vi "CmdParse_3.vi"(8 "error in (no error)":errorcluster, 9 "Read Buffer":string, 10 "Node Id":u8, 11 "Socket Id":u8) -> (0 "error out":errorcluster)   [LabVIEW 2011]
uses:
  Enumerator/CmdType.ctl
  Variable/gSIM.vi
  DLL/Certificate_03.vi
  Variable/gSEL.vi
  Look-up/Password/PSW_03.vi
  Queue/Door_03.vi
  Interface/SockeHook/Hook_03.vi
panel:
  in  "KeyPass":bool
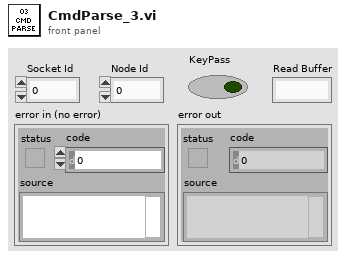
[diagram p1: front panel]
types:
  T1 = enum16{"Open", "R", "W", "R->W", "W->R", "Close"}
  T2 = typedef "CmdType.ctl" = enum16{"GetEventLog", "DelTransaction", "InvalidMessage", "RelayControl", "RelayOff", "RelayOn", "VaildMessage", "EventPolling", "StoppingWaiting", "PromptKeying-in"}
  T3 = enum16{"Open", "Verify", "Password", "Log", "Close"}
  T4 = enum16{"Obtain", "Enqueue", "Dequeue", "Release"}
  T5 = cluster{"unsigned byte array":u8[], "Socket Id":u8, u8}
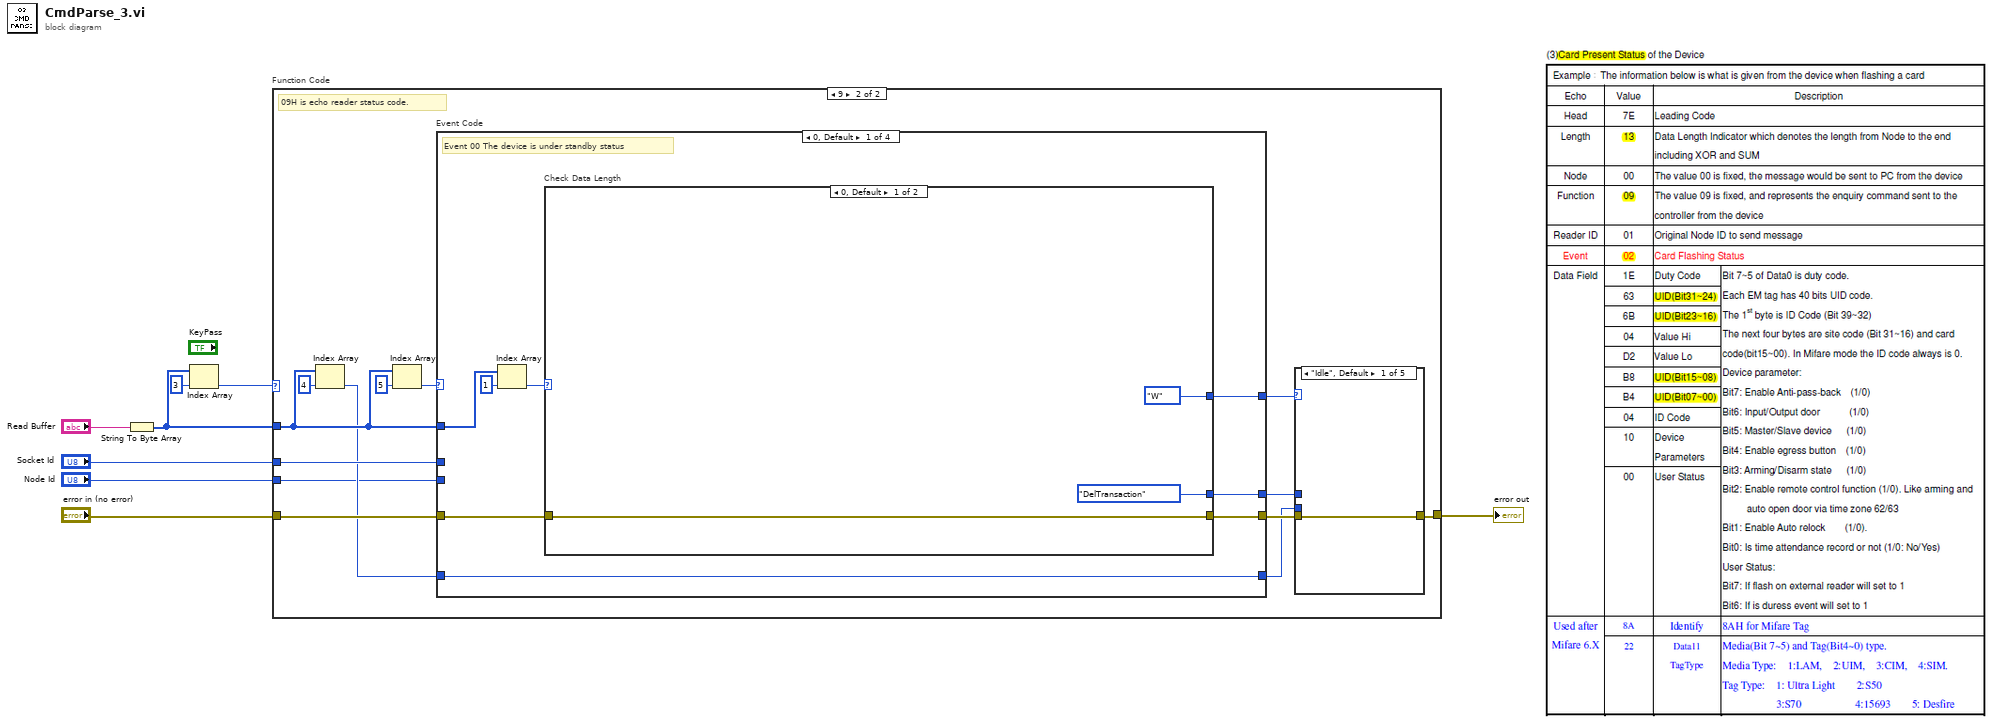
[diagram p0: block diagram]
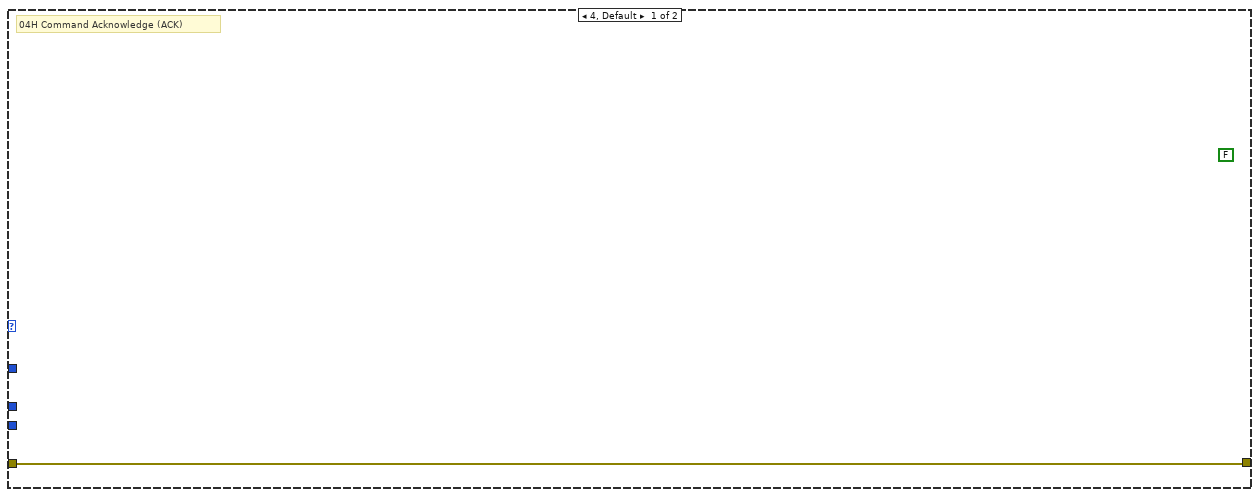
[diagram p2: hidden frame]
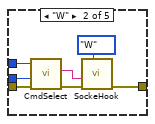
[diagram p3: hidden frame]
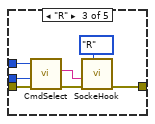
[diagram p4: hidden frame]
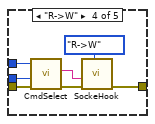
[diagram p5: hidden frame]
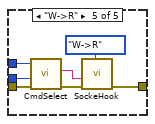
[diagram p6: hidden frame]
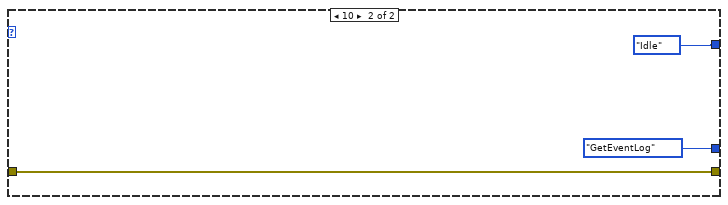
[diagram p7: hidden frame]
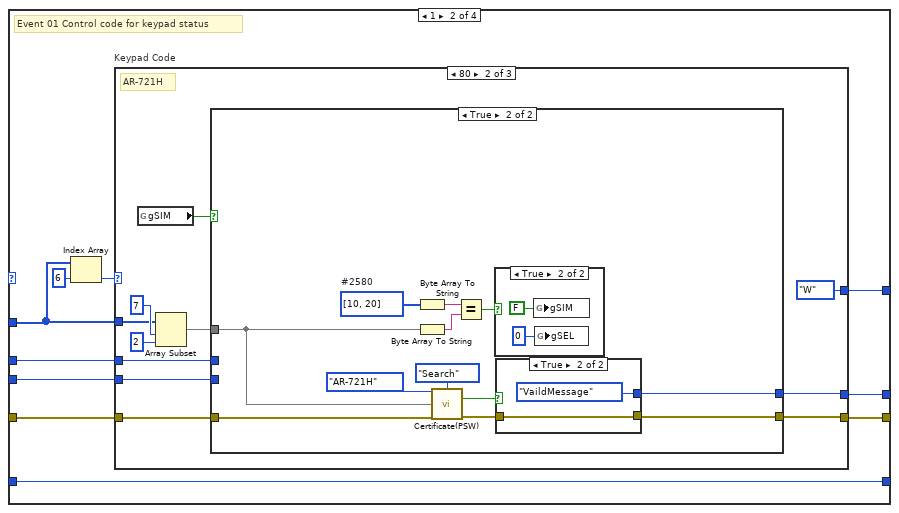
[diagram p8: hidden frame]
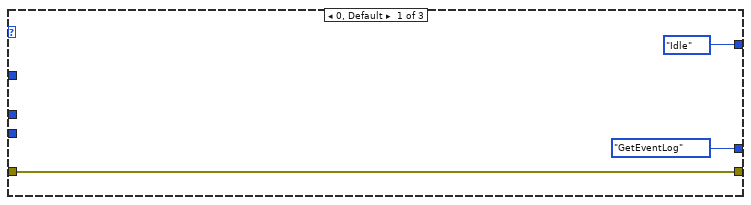
[diagram p9: hidden frame]
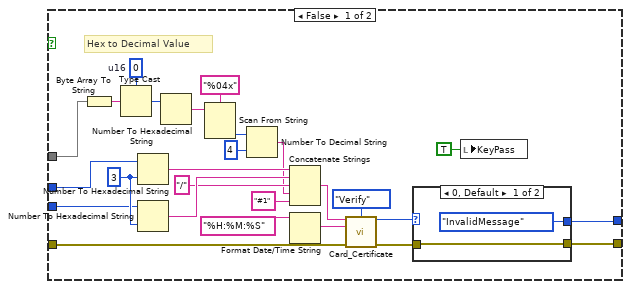
[diagram p10: hidden frame]
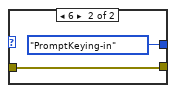
[diagram p11: hidden frame]
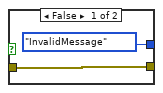
[diagram p12: hidden frame]
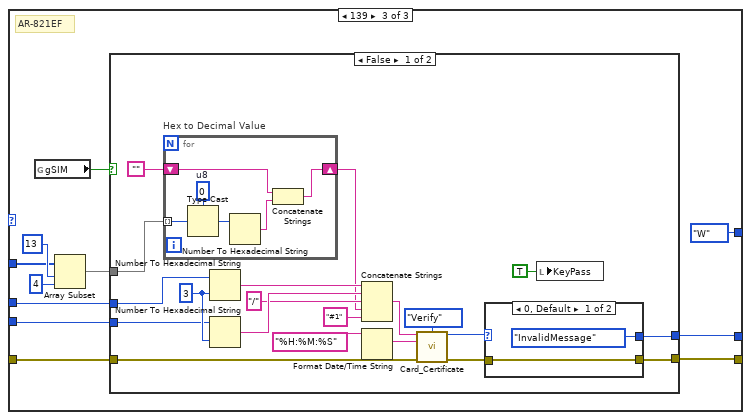
[diagram p14: hidden frame]
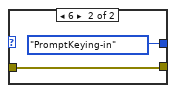
[diagram p15: hidden frame]
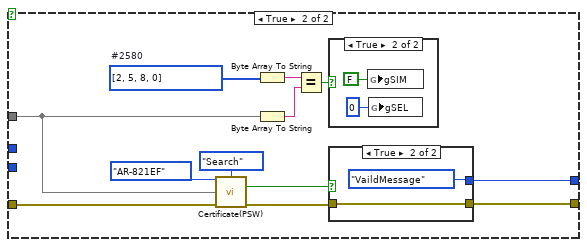
[diagram p16: hidden frame]
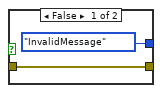
[diagram p17: hidden frame]
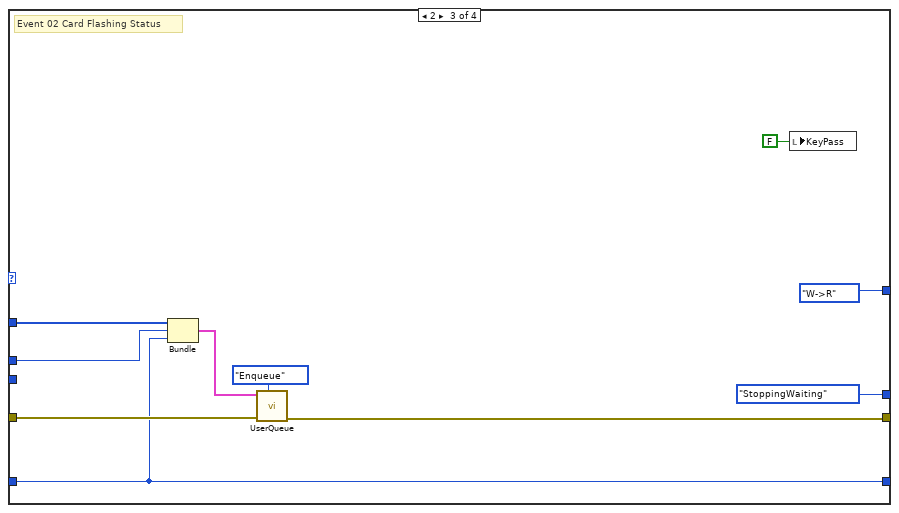
[diagram p19: hidden frame]
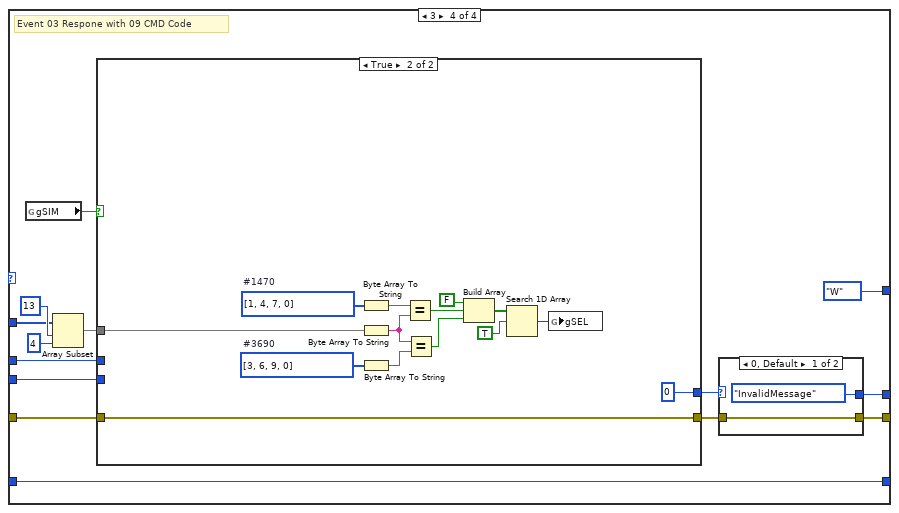
[diagram p20: hidden frame]
diagram:
  n1 = String To Byte Array(string="Read Buffer") -> (unsigned byte array=w2:u8[])
  n2 = Index Array(array=w2, index=3) -> (element=w5:u8)
  n3 = case "Function Code" shown="9" w5 {
    tunnel: "error in (no error)" -> [w9 w22]
    tunnel: [w9 w14] -> w8
    tunnel: w2 -> [_ w20]
    tunnel: "Socket Id" -> [_ w19]
    tunnel: "Node Id" -> [_ w10]
    frame 4, Default {
      (unwired) FALSE
      # "04H Command Acknowledge (ACK)"
    }
    frame 9 {
      # "09H is echo reader status code."
      n4 = Index Array(array=w20, index=4) -> (element=w16:u8)
      n5 = Index Array(array=w20, index=5) -> (element=w17:u8)
      n6 = case "Event Code" shown="0, Default" w17 {
        tunnel: w22 -> [w59 w75 w199 w212]
        tunnel: w16 -> [w52 w68 w198 w216]
        tunnel: [w58 w74 w206 w218] -> w15
        tunnel: w20 -> [w55 w71 w204 w215]
        tunnel: w19 -> [_ w67 w203 w208]
        tunnel: [w52 w68 w198 w216] -> w13
        tunnel: [w54 w70 CmdType."StoppingWaiting" ("CmdType") w214] -> w12
        tunnel: [w53 w69 enum16{"Idle", "R", "W", "R->W", "W->R"}."W->R" ("Mode") enum16{"Idle", "R", "W", "R->W", "W->R"}."W" ("Mode")] -> w11
        tunnel: w10 -> [_ w66 _ w207]
        frame 0, Default {
          # "Event 00 The device is under standby status"
          n7 = Index Array(array=w55, index=1) -> (element=w56:u8)
          n8 = case "Check Data Length" shown="0, Default" w56 {
            tunnel: w59 -> [w62 w65]
            tunnel: [w62 w65] -> w58
            tunnel: [CmdType."DelTransaction" ("CmdType") CmdType."GetEventLog" ("CmdType")] -> w54
            tunnel: [enum16{"Idle", "R", "W", "R->W", "W->R"}."W" ("Mode") enum16{"Idle", "R", "W", "R->W", "W->R"}."Idle" ("Mode")] -> w53
            frame 0, Default {
            }
            frame 10 {
            }
          }
        }
        frame 1 {
          # "Event 01 Control code for keypad status"
          n9 = Index Array(array=w71, index=6) -> (element=w72:u8)
          n10 = case "Keypad Code" shown="80" w72 {
            tunnel: w75 -> [w78 w82 w142]
            tunnel: [w78 w83 w141] -> w74
            tunnel: w71 -> [_ w87 w146]
            tunnel: [CmdType."GetEventLog" ("CmdType") w81 w140] -> w70
            tunnel: [enum16{"Idle", "R", "W", "R->W", "W->R"}."Idle" ("Mode") enum16{"Idle", "R", "W", "R->W", "W->R"}."W" ("Mode") enum16{"Idle", "R", "W", "R->W", "W->R"}."W" ("Mode")] -> w69
            tunnel: w67 -> [_ w80 w139]
            tunnel: w66 -> [_ w79 w138]
            frame 0, Default {
            }
            frame 128 {
              # "AR-721H"
              n11 = global read "gSIM.vi" "gSIM"() -> (w85:bool)
              n12 = Array Subset(array=w87, index=7, length=2) -> (w84:u8[])
              n13 = case shown="True" w85 {
                tunnel: w84 -> [w98 w120]
                tunnel: [w113 w123] -> w83
                tunnel: w82 -> [w114 w122]
                tunnel: [w110 w121] -> w81
                tunnel: w80 -> [w103 _]
                tunnel: w79 -> [w102 _]
                frame False {
                  w97 = u16 0  # u16
                  w106 = i16 3 ("width (-)")
                  # "Hex to Decimal Value"
                  n14 = Byte Array To String(unsigned byte array=w98) -> (string=w99:string)
                  n15 = Type Cast(type=w97, x=w99) -> (*(type *) &x=w96:u16)
                  n16 = Number To Hexadecimal String(1:w106, 2:w103) -> (0:w109:string)
                  n17 = Number To Hexadecimal String(1:w106, 2:w102) -> (0:w108:string)
                  n18 = Number To Hexadecimal String(2:w96) -> (0:w95:string)  [unwired: 1 in]
                  n19 = Scan From String(format string="%04x", input string=w95) -> (output 1=w93:i32)  [unwired: 2 in, 4 out]
                  n20 = Number To Decimal String(number=w93, width (-)=i16 4) -> (decimal integer string=w92:string)
                  n21 = Concatenate Strings(w109, w108, "/" ("string"), w92, "#1" ("string")) -> (w100:string)
                  n22 = Format Date/Time String(time format string (%c)="%H:%M:%S") -> (date/time string=w101:string)  [unwired: 2 in]
                  n23 = call-poly "Card_Certificate.vi"("CardNumber"=w100, "DB"=T3."Verify", "Time"=w101, "error in"=w114) -> ("Certificate"=w111:u8, "error out"=w112:errorcluster)  [unwired: 10 in]
                  n24 = case shown="0, Default" w111 {
                    tunnel: w112 -> [w117 w119]
                    tunnel: [w117 w119] -> w113
                    tunnel: [CmdType."InvalidMessage" ("CmdType") CmdType."PromptKeying-in" ("CmdType")] -> w110
                    frame 0, Default {
                    }
                    frame 6 {
                    }
                  }
                  n25 = local write "KeyPass"(TRUE ("KeyPass")) -> ()
                }
                frame True {
                  w130 = u8[] [10, 20]  # #2580
                  n26 = Byte Array To String(unsigned byte array=w130) -> (string=w131:string)
                  n27 = Byte Array To String(unsigned byte array=w120) -> (string=w129:string)
                  n28 = call-poly "Certificate(PSW).vi"("type"=enum16{"AR-721H", "AR-821EF"}."AR-721H", "select"=enum16{"Setup", "Search", "Release"}."Search", "key"=w120, "error in"=w122) -> ("found"=w127:bool, "error out"=w126:errorcluster)  [unwired: 9 in, 1 out]
                  n29 = Equal?(x=w131, y=w129) -> (x = y?=w128:bool)
                  n30 = case shown="True" w128 {
                    frame False {
                    }
                    frame True {
                      n31 = global write "gSIM.vi" "gSIM"(FALSE ("gSIM")) -> ()
                      n32 = global write "gSEL.vi" "gSEL"(0 ("gSEL")) -> ()
                    }
                  }
                  n33 = case shown="True" w127 {
                    tunnel: w126 -> [w133 w135]
                    tunnel: [w133 w135] -> w123
                    tunnel: [CmdType."InvalidMessage" ("CmdType") CmdType."VaildMessage" ("CmdType")] -> w121
                    frame False {
                    }
                    frame True {
                    }
                  }
                }
              }
            }
            frame 139 {
              # "AR-821EF"
              n34 = global read "gSIM.vi" "gSIM"() -> (w144:bool)
              n35 = Array Subset(array=w146, index=13, length=4) -> (w143:u8[])
              n36 = case shown="False" w144 {
                tunnel: w143 -> [w158 w179]
                tunnel: w142 -> [w154 w182]
                tunnel: [w162 w181] -> w141
                tunnel: [w156 w180] -> w140
                tunnel: w139 -> [w161 _]
                tunnel: w138 -> [w160 _]
                frame False {
                  w165 = i16 3 ("width (-)")
                  n37 = for "Hex to Decimal Value" {
                    shift-right: [w171] -> w157
                    shift-left: "" -> [w170]
                    tunnel: w158 -> [w169] mode=indexing
                    w173 = u8 0  # u8
                    n38 = Type Cast(type=w173, x=w169) -> (*(type *) &x=w174:u8)
                    n39 = Number To Hexadecimal String(2:w174) -> (0:w172:string)  [unwired: 1 in]
                    n40 = Concatenate Strings(w170, w172) -> (w171:string)
                  }
                  n41 = Number To Hexadecimal String(1:w165, 2:w161) -> (0:w168:string)
                  n42 = Number To Hexadecimal String(1:w165, 2:w160) -> (0:w167:string)
                  n43 = Concatenate Strings(w168, w167, "/" ("string"), w157, "#1" ("string")) -> (w151:string)
                  n44 = Format Date/Time String(time format string (%c)="%H:%M:%S") -> (date/time string=w150:string)  [unwired: 2 in]
                  n45 = call-poly "Card_Certificate.vi"("CardNumber"=w151, "DB"=T3."Verify", "Time"=w150, "error in"=w154) -> ("Certificate"=w152:u8, "error out"=w153:errorcluster)  [unwired: 10 in]
                  n46 = case shown="0, Default" w152 {
                    tunnel: w153 -> [w176 w178]
                    tunnel: [w176 w178] -> w162
                    tunnel: [CmdType."InvalidMessage" ("CmdType") CmdType."PromptKeying-in" ("CmdType")] -> w156
                    frame 0, Default {
                    }
                    frame 6 {
                    }
                  }
                  n47 = local write "KeyPass"(TRUE ("KeyPass")) -> ()
                }
                frame True {
                  w188 = u8[] [2, 5, 8, 0]  # #2580
                  n48 = call-poly "Certificate(PSW).vi"("type"=enum16{"AR-721H", "AR-821EF"}."AR-821EF", "select"=enum16{"Setup", "Search", "Release"}."Search", "key"=w179, "error in"=w182) -> ("found"=w185:bool, "error out"=w184:errorcluster)  [unwired: 9 in, 1 out]
                  n49 = Byte Array To String(unsigned byte array=w188) -> (string=w190:string)
                  n50 = Byte Array To String(unsigned byte array=w179) -> (string=w189:string)
                  n51 = Equal?(x=w190, y=w189) -> (x = y?=w187:bool)
                  n52 = case shown="True" w187 {
                    frame False {
                    }
                    frame True {
                      n53 = global write "gSIM.vi" "gSIM"(FALSE ("gSIM")) -> ()
                      n54 = global write "gSEL.vi" "gSEL"(0 ("gSEL")) -> ()
                    }
                  }
                  n55 = case shown="True" w185 {
                    tunnel: w184 -> [w192 w194]
                    tunnel: [w192 w194] -> w181
                    tunnel: [CmdType."InvalidMessage" ("CmdType") CmdType."VaildMessage" ("CmdType")] -> w180
                    frame False {
                    }
                    frame True {
                    }
                  }
                }
              }
            }
          }
        }
        frame 2 {
          # "Event 02 Card Flashing Status"
          n56 = Bundle("unsigned byte array"=w204, "Socket Id"=w203, w198) -> (w202:T5)  [unwired: 1 in]
          n57 = call-poly "UserQueue.vi"("Mode"=T4."Enqueue", "error in (no error)"=w199, "Queue In"=w202) -> ("error out"=w206:errorcluster)  [unwired: 7 in, 1 out]
          n58 = local write "KeyPass"(FALSE) -> ()
        }
        frame 3 {
          # "Event 03 Respone with 09 CMD Code"
          n59 = global read "gSIM.vi" "gSIM"() -> (w213:bool)
          n60 = Array Subset(array=w215, index=13, length=4) -> (w209:u8[])
          n61 = case shown="True" w213 {
            tunnel: w212 -> [w227 w268]
            tunnel: [w226 w268] -> w211
            tunnel: [w225 u8 0 ("Certificate")] -> w210
            tunnel: w209 -> [w224 w267]
            tunnel: w208 -> [w223 _]
            tunnel: w207 -> [w222 _]
            frame False {
              n62 = local read "KeyPass"() -> (w221:bool)
              n63 = case shown="False" w221 {
                tunnel: w227 -> [w230 w258]
                tunnel: [w231 w257] -> w226
                tunnel: [w228 w256] -> w225
                tunnel: w224 -> [w229 w255]
                tunnel: w223 -> [_ w254]
                tunnel: w222 -> [_ w253]
                frame False {
                  n64 = for "Number To Decimal String" {
                    shift-right: [w240] -> w233
                    shift-left: "" -> [w239]
                    tunnel: w229 -> [w237] mode=indexing
                    n65 = Number To Decimal String(number=w237, width (-)=i16 1) -> (decimal integer string=w238:string)
                    n66 = Concatenate Strings(w239, w238) -> (w240:string)
                  }
                  n67 = Concatenate Strings(";" ("string"), w233) -> (w234:string)
                  n68 = call-poly "Card_Certificate.vi"("DB"=T3."Password", "Password"=w234, "error in"=w230) -> ("Certificate"=w228:u8, "error out"=w231:errorcluster)  [unwired: 11 in]
                }
                frame True {
                  w248 = i16 3 ("width (-)")
                  n69 = for "Number To Decimal String" {
                    shift-right: [w262] -> w246
                    shift-left: "" -> [w261]
                    tunnel: w255 -> [w259] mode=indexing
                    n70 = Number To Decimal String(number=w259, width (-)=i16 1) -> (decimal integer string=w260:string)
                    n71 = Concatenate Strings(w261, w260) -> (w262:string)
                  }
                  n72 = Number To Hexadecimal String(1:w248, 2:w254) -> (0:w251:string)
                  n73 = Number To Hexadecimal String(1:w248, 2:w253) -> (0:w250:string)
                  n74 = Concatenate Strings(w251, w250, "/" ("string"), w246, "#2" ("string")) -> (w243:string)
                  n75 = Format Date/Time String(time format string (%c)="%H:%M:%S") -> (date/time string=w242:string)  [unwired: 2 in]
                  n76 = call-poly "Card_Certificate.vi"("CardNumber"=w243, "DB"=T3."Verify", "Time"=w242, "error in"=w258) -> ("Certificate"=w256:u8, "error out"=w257:errorcluster)  [unwired: 10 in]
                }
              }
            }
            frame True {
              w274 = u8[] [3, 6, 9, 0]  # #3690
              w270 = u8[] [1, 4, 7, 0]  # #1470
              n77 = Byte Array To String(unsigned byte array=w270) -> (string=w273:string)
              n78 = Byte Array To String(unsigned byte array=w267) -> (string=w265:string)
              n79 = Byte Array To String(unsigned byte array=w274) -> (string=w266:string)
              n80 = Equal?(x=w273, y=w265) -> (x = y?=w272:bool)
              n81 = Equal?(x=w265, y=w266) -> (x = y?=w271:bool)
              n82 = Build Array(FALSE ("element"), w272, w271) -> (w276:bool[])
              n83 = Search 1D Array(1D array=w276, element=TRUE) -> (index of element=w275:i32)  [unwired: 1 in]
              n84 = global write "gSEL.vi" "gSEL"(w275) -> ()
            }
          }
          n85 = case shown="0, Default" w210 {
            tunnel: w211 -> [w279 w281]
            tunnel: [w279 w281] -> w218
            tunnel: [CmdType."InvalidMessage" ("CmdType") CmdType."VaildMessage" ("CmdType")] -> w214
            frame 0, Default {
            }
            frame 1 {
            }
          }
        }
      }
      n86 = case shown="\"Idle\", Default" w11 {
        tunnel: w15 -> [w23 w27 w34 w41 w48]
        tunnel: [w23 w26 w33 w40 w47] -> w14
        tunnel: w13 -> [_ w25 w32 w39 w46]
        tunnel: w12 -> [_ w24 w31 w38 w45]
        frame "Idle", Default {
        }
        frame "W" {
          n87 = call "CmdSelect.vi"("error in (no error)"=w27, "Node Id"=w25, "Cmd Type"=w24) -> ("error out"=w29:errorcluster, "Cmd Str"=w28:string)  [unwired: 7 in]
          n88 = call-poly "SockeHook.vi"("Mode"=T1."W", "error in (no error)"=w29, "data in"=w28) -> ("error out"=w26:errorcluster)  [unwired: 7 in, 1 out]
        }
        frame "R" {
          n89 = call "CmdSelect.vi"("error in (no error)"=w34, "Node Id"=w32, "Cmd Type"=w31) -> ("error out"=w36:errorcluster, "Cmd Str"=w35:string)  [unwired: 7 in]
          n90 = call-poly "SockeHook.vi"("Mode"=T1."R", "error in (no error)"=w36, "data in"=w35) -> ("error out"=w33:errorcluster)  [unwired: 7 in, 1 out]
        }
        frame "R->W" {
          n91 = call "CmdSelect.vi"("error in (no error)"=w41, "Node Id"=w39, "Cmd Type"=w38) -> ("error out"=w43:errorcluster, "Cmd Str"=w42:string)  [unwired: 7 in]
          n92 = call-poly "SockeHook.vi"("Mode"=T1."R->W", "error in (no error)"=w43, "data in"=w42) -> ("error out"=w40:errorcluster)  [unwired: 7 in, 1 out]
        }
        frame "W->R" {
          n93 = call "CmdSelect.vi"("error in (no error)"=w48, "Node Id"=w46, "Cmd Type"=w45) -> ("error out"=w50:errorcluster, "Cmd Str"=w49:string)  [unwired: 7 in]
          n94 = call-poly "SockeHook.vi"("Mode"=T1."W->R", "error in (no error)"=w50, "data in"=w49) -> ("error out"=w47:errorcluster)  [unwired: 7 in, 1 out]
        }
      }
    }
  }
  "error out" <- w8
